vi "Vacuum_System.vi"() -> ()   [LabVIEW 2018]
uses:
  InstrumentStatusLib/com.insstat.lvlib
panel:
  out "?":bool
  out "?":bool
  out "?":bool
  out "?":string
  out "?":string
  out "?":bool
  out "?":bool
  out "?":bool
  out "?":bool
  out "?":bool
  out "?":string
  out "?":string
  out "?":string
  out "?":bool
  out "?":string
  out "?":bool
  out "?":bool
  out "?":bool
  out "?":bool
  out "?":bool
  out "?":string
  out "?":string
  out "?":string
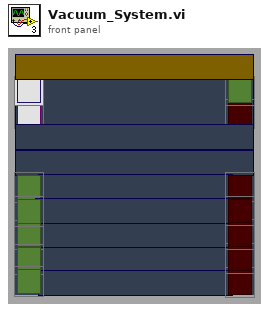
[diagram p1: front panel]
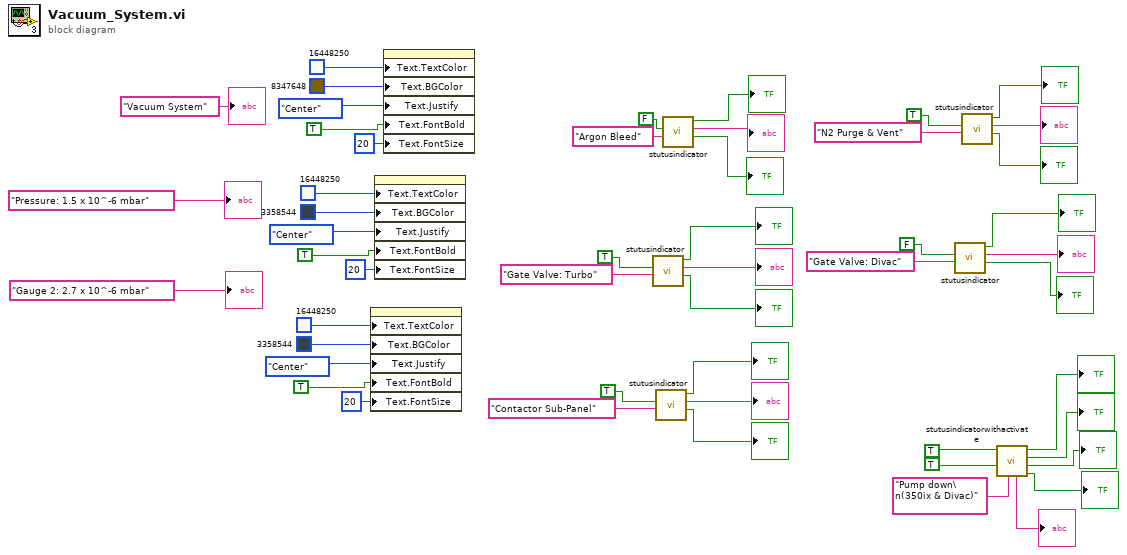
[diagram p0: block diagram]
diagram:
  n1 = property class="Str"("Text.TextColor"=u32 16448250, "Text.BGColor"=u32 3358544, "Text.Justify"=enum16{"Left", "Center", "Right"}."Center" ("Text.Justification"), "Text.FontBold"=TRUE ("Text.Font:Bold"), "Text.FontSize"=u32 20 ("Text.Font:Size")) -> ()  [unwired: 2 in, 2 out]
  n2 = property class="Str"("Text.TextColor"=u32 16448250, "Text.BGColor"=u32 3358544, "Text.Justify"=enum16{"Left", "Center", "Right"}."Center" ("Text.Justification"), "Text.FontBold"=TRUE ("Text.Font:Bold"), "Text.FontSize"=u32 20 ("Text.Font:Size")) -> ()  [unwired: 2 in, 2 out]
  n3 = property class="Str"("Text.TextColor"=u32 16448250, "Text.BGColor"=u32 8347648, "Text.Justify"=enum16{"Left", "Center", "Right"}."Center" ("Text.Justification"), "Text.FontBold"=TRUE ("Text.Font:Bold"), "Text.FontSize"=u32 20 ("Text.Font:Size")) -> ()  [unwired: 2 in, 2 out]
  n4 = call "stutusindicator.vi"("String"="Gate Valve: Turbo", "Boolean"=TRUE) -> (1:→"?":bool, 2:→"?":string, 3:→"?":bool)  [unwired: 7 in]
  n5 = call "stutusindicator.vi"("String"="Contactor Sub-Panel", "Boolean"=TRUE) -> (1:→"?":bool, 2:→"?":string, 3:→"?":bool)  [unwired: 7 in]
  n6 = call "stutusindicator.vi"("String"="Argon Bleed", "Boolean"=FALSE) -> (1:→"?":bool, 2:→"?":string, 3:→"?":bool)  [unwired: 7 in]
  n7 = call "stutusindicator.vi"("String"="Gate Valve: Divac", "Boolean"=FALSE) -> (1:→"?":bool, 2:→"?":string, 3:→"?":bool)  [unwired: 7 in]
  n8 = call "stutusindicator.vi"("String"="N2 Purge & Vent", "Boolean"=TRUE) -> (1:→"?":bool, 2:→"?":string, 3:→"?":bool)  [unwired: 7 in]
  n9 = call "stutusindicatorwithactivate.vi"("String"="Pump down\n(350ix & Divac)", "Power"=TRUE, "Activate"=TRUE) -> (0:→"?":bool, 1:→"?":bool, 2:→"?":bool, 3:→"?":bool, 4:→"?":string)  [unwired: 4 in]
  "?" <- "Vacuum System" ("String")
  "?" <- "Pressure: 1.5 x 10^-6 mbar"
  "?" <- "Gauge 2: 2.7 x 10^-6 mbar"
